vi "Add Parameter.vi"(8 "error in":errorcluster, 10 "parameter configuration":T1 {"direction" items=["incoming", "outgoing"]}, 11 "label in":refnum<k24>) -> (0 "error out":errorcluster, 2 "new parameter":refnum<k24>, 3 "label out":refnum<k24>)   [LabVIEW 2020, in "Ballard_429_Parameter_ni.lvlib"]
uses:
  Ballard_429_Parameter_ni.lvlib
  _tyedefs/parameter_type.ctl
  C:/Users/Administrator/Desktop/GIT/Ballard-Arinc-429-XML-Generator/Source/Assemblies/Ballard_429_Parameter_ni/bin/Debug/Ballard_429_Parameter_ni.dll
  Assemblies/Ballard_429_Parameter_ni/bin/Debug/Ballard_429_Parameter_ni.dll
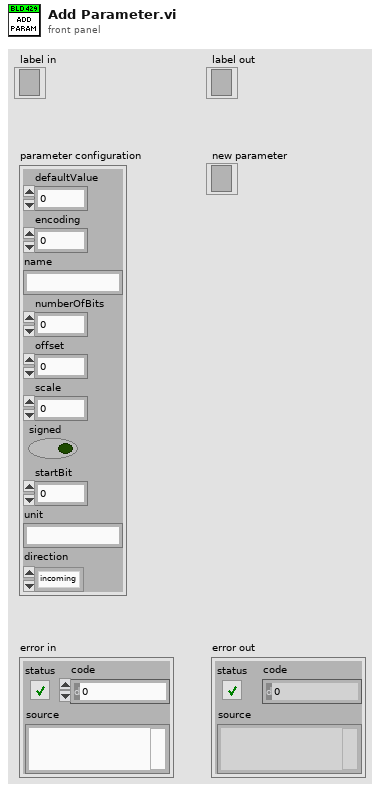
[diagram p1: front panel]
types:
  T1 = typedef "Ballard_429_Parameter_ni.lvlib/parameter_type.ctl" = cluster{"defaultValue":dbl, "encoding":i32, "name":string, "numberOfBits":i32, "offset":dbl, "scale":dbl, "signed":bool, "startBit":i32, "unit":string, "direction":i32}
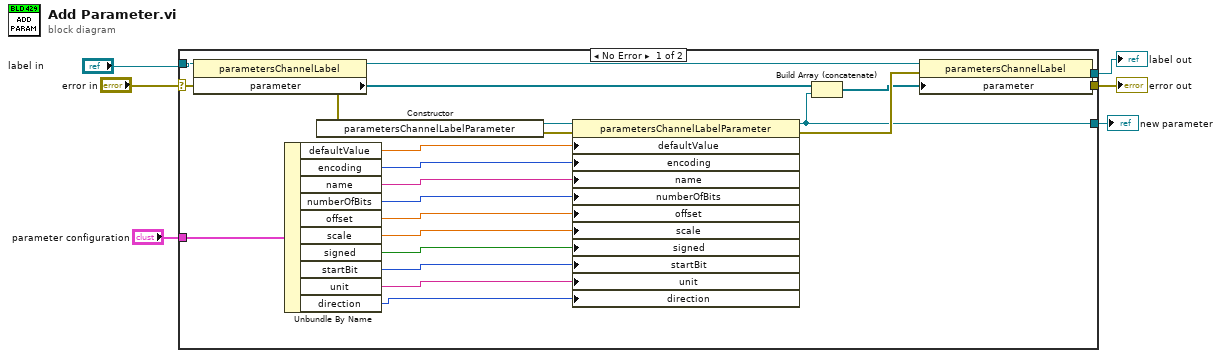
[diagram p0: block diagram]
diagram:
  n1 = case shown="No Error" "error in" {
    selector: "error in" -> [w28 w30]
    tunnel: [w24 w31] -> w6
    tunnel: [w23 w30] -> w5
    tunnel: "label in" -> [w29 w31]
    tunnel: [w9 _] -> w1
    tunnel: "parameter configuration" -> [w19 _]
    frame No Error {
      n2 = property class="parametersChannelLabel"(reference=w29, error in=w28) -> (reference out=w25:refnum<k24>, error out=w26:errorcluster, "parameter"=w27:refnum<k24>[])
      n3 = Unbundle By Name(w19) -> ("defaultValue"=w18:dbl, "encoding"=w17:i32, "name"=w16:string, "numberOfBits"=w15:i32, "offset"=w14:dbl, "scale"=w13:dbl, "signed"=w12:bool, "startBit"=w11:i32, "unit"=w10:string, "direction"=w7:i32)
      n4 = constructor class="parametersChannelLabelParameter"(error in=w26) -> (reference out=w22:refnum<k24>, error out=w21:errorcluster)  [unwired: 2 in, 1 out]
      n5 = property class="parametersChannelLabelParameter"(reference=w22, error in=w21, "defaultValue"=w18, "encoding"=w17, "name"=w16, "numberOfBits"=w15, "offset"=w14, "scale"=w13, "signed"=w12, "startBit"=w11, "unit"=w10, "direction"=w7) -> (reference out=w9:refnum<k24>, error out=w20:errorcluster)
      n6 = Build Array (concatenate)(w27, w9) -> (w8:refnum<k24>[])
      n7 = property class="parametersChannelLabel"(reference=w25, error in=w20, "parameter"=w8) -> (reference out=w24:refnum<k24>, error out=w23:errorcluster)
    }
    frame Error {
    }
  }
  "label out" <- w6
  "error out" <- w5
  "new parameter" <- w1
